vi "Deallocate Block.vi"   [LabVIEW 2016, in "GE 5565PIORC.lvclass"]
uses:
  GE 5565PIORC.lvclass
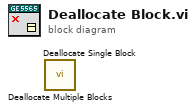
[diagram p0: block diagram]
diagram:
  n1 = call "Deallocate Multiple Blocks.vi"() -> ()  [unwired: 10 in, 2 out]
  n2 = call "Deallocate Single Block.vi"() -> ()  [unwired: 10 in, 2 out]
